vi "RampDrive.vi"(2 "Buttons":T2, 3 "Axes":T1) -> (0 "Right Speed":dbl, 1 "Left Speed":dbl)   [LabVIEW 2011]
uses:
  <vilib>/Rock Robotics/WPI/Joystick/WPI_JoystickButtonState.ctl
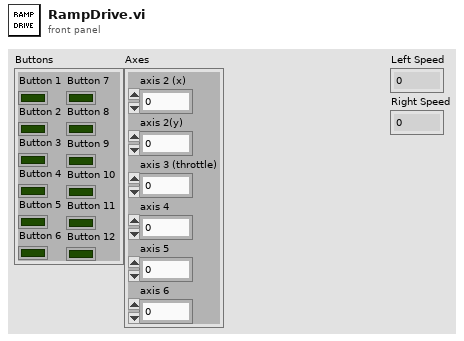
[diagram p1: front panel]
types:
  T1 = cluster{"axis 2 (x)":dbl, "axis 2(y)":dbl, "axis 3 (throttle)":dbl, "axis 4":dbl, "axis 5":dbl, "axis 6":dbl}
  T2 = typedef "WPI_JoystickButtonState.ctl" = cluster{"Button 1":bool, "Button 2":bool, "Button 3":bool, "Button 4":bool, "Button 5":bool, "Button 6":bool, "Button 7":bool, "Button 8":bool, "Button 9":bool, "Button 10":bool, "Button 11":bool, "Button 12":bool}
  T3 = cluster{"Button 5":bool, "Button 6":bool, "Button 7":bool, "Button 8":bool}
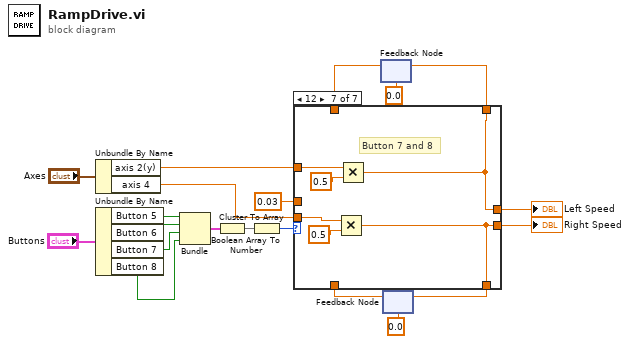
[diagram p0: block diagram]
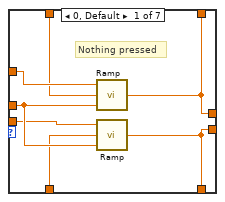
[diagram p2: hidden frame]
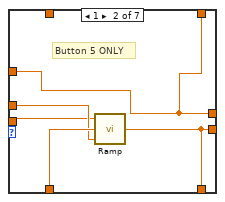
[diagram p3: hidden frame]
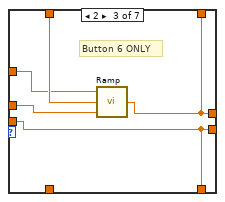
[diagram p4: hidden frame]
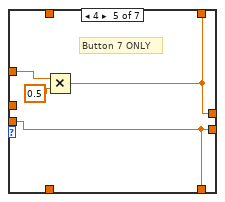
[diagram p6: hidden frame]
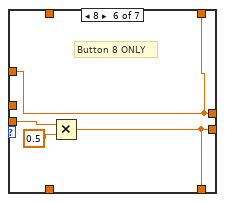
[diagram p7: hidden frame]
diagram:
  n1 = Unbundle By Name("Axes") -> ("axis 2(y)"=w2:dbl, "axis 4"=w1:dbl)
  n2 = Unbundle By Name("Buttons") -> ("Button 5"=w19:bool, "Button 6"=w18:bool, "Button 7"=w17:bool, "Button 8"=w16:bool)
  n3 = Bundle("Button 5"=w19, "Button 6"=w18, "Button 7"=w17, "Button 8"=w16) -> (w14:T3)  [unwired: 1 in]
  n4 = Cluster To Array(cluster=w14) -> (array=w15:bool[])
  n5 = Boolean Array To Number(Boolean array=w15) -> (number=w12:u32)
  n6 = feedback #1(0.0 ("axis 2(y)")) -> (w10:dbl)
  n7 = feedback #2(0.0 ("axis 2(y)")) -> (w4:dbl)
  n8 = case shown="12" w12 {
    tunnel: w2 -> [w27 w29 w36 w38 w43 w47 w49]
    tunnel: 0.03 ("Speed increment") -> [w24 w30 w34 _ _ _ _]
    tunnel: [w25 w29 w35 w38 w41 w47 w48] -> w8
    tunnel: w10 -> [w26 _ w37 _ _ _ _]
    tunnel: [w25 w29 w35 w38 w41 w47 w48] -> w7
    tunnel: [w22 w31 w33 w39 w40 w44 w51] -> w6
    tunnel: w4 -> [w23 w32 _ _ _ _ _]
    tunnel: [w22 w31 w33 w39 w40 w44 w51] -> w3
    tunnel: w1 -> [w21 w28 w33 w39 w40 w46 w53]
    frame 0, Default {
      # "Nothing pressed"
      n9 = call "Ramp.vi"("Speed increment"=w24, "last speed"=w26, "Joystick speed"=w27) -> ("speed setting"=w25:dbl)
      n10 = call "Ramp.vi"("Speed increment"=w24, "last speed"=w23, "Joystick speed"=w21) -> ("speed setting"=w22:dbl)
    }
    frame 1 {
      # "Button 5 ONLY"
      n11 = call "Ramp.vi"("Speed increment"=w30, "last speed"=w32, "Joystick speed"=w28) -> ("speed setting"=w31:dbl)
    }
    frame 2 {
      # "Button 6 ONLY"
      n12 = call "Ramp.vi"("Speed increment"=w34, "last speed"=w37, "Joystick speed"=w36) -> ("speed setting"=w35:dbl)
    }
    frame 3 {
      # "Button 5 and 6"
    }
    frame 4 {
      # "Button 7 ONLY"
      n13 = Multiply(x=w43, y=0.5) -> (x*y=w41:dbl)
    }
    frame 8 {
      # "Button 8 ONLY"
      n14 = Multiply(x=w46, y=0.5) -> (x*y=w44:dbl)
    }
    frame 12 {
      # "Button 7 and 8"
      n15 = Multiply(x=w53, y=0.5) -> (x*y=w51:dbl)
      n16 = Multiply(x=w49, y=0.5) -> (x*y=w48:dbl)
    }
  }
  "Left Speed" <- w8
  "Right Speed" <- w6
  n17 = feedback-in #1(w7) -> ()
  n18 = feedback-in #2(w3) -> ()
